vi "Example Remote Callback.vi"() -> ()   [LabVIEW 2013]
uses:
  C:/tf/play/labview/Tinkerforge.dll
  Tinkerforge.dll
panel:
  out "repeats":i32
  out "switchTo":i32
  out "receiverCode":u8
  out "houseCode":u8
  in  "stop":bool
  in  "uid":string="abc"
  in  "port":i32=4223
  in  "host":string="localhost"
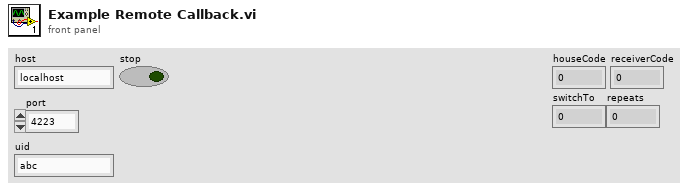
[diagram p1: front panel]
types:
  T1 = cluster{"houseCode":u8, "receiverCode":u8, "repeats":i32, "switchTo":i32}
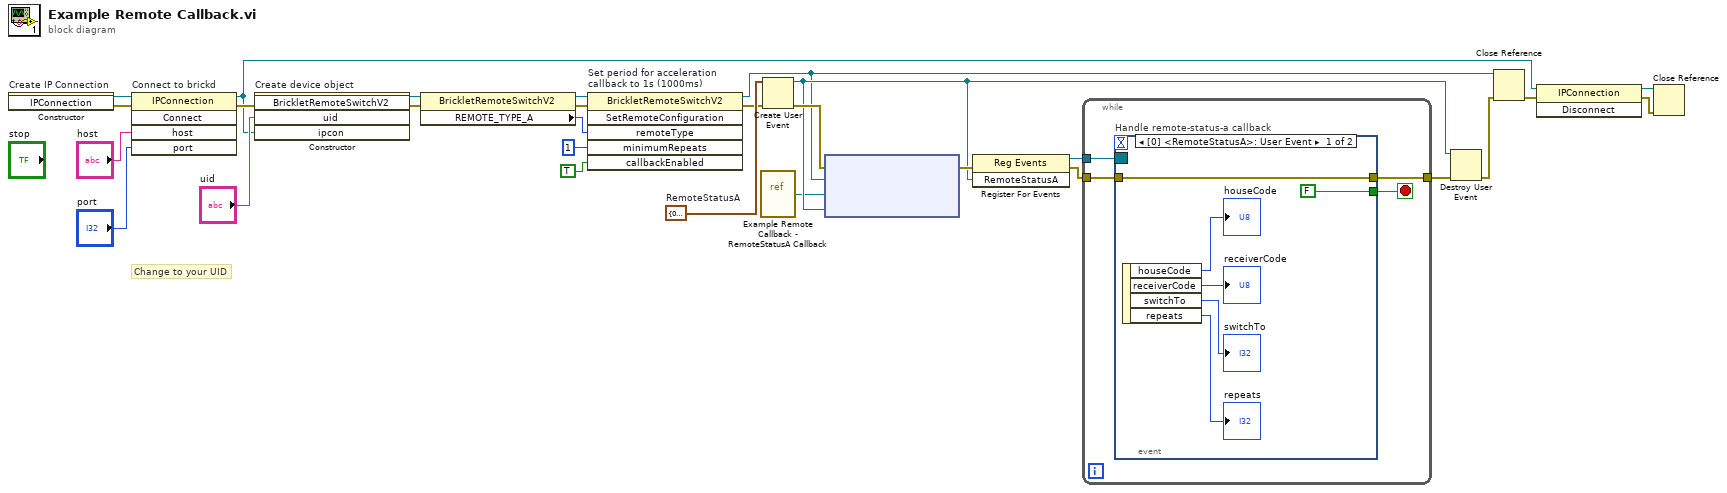
[diagram p0: block diagram]
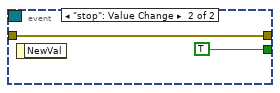
[diagram p2: hidden frame]
diagram:
  w12 = T1 {"houseCode"=0, "receiverCode"=0, "repeats"=0, "switchTo"=0}  # RemoteStatusA
  # "Change to your UID"
  n1 = constructor on="Create IP Connection" class="IPConnection"() -> (reference out=w28:refnum<k24>, error out=w9:errorcluster)  [unwired: 3 in, 1 out]
  n2 = invoke on="Connect to brickd" class="IPConnection" method="Connect"(reference=w28, error in=w9, "host"="host", "port"="port") -> (reference out=w21:refnum<k24>, error out=w24:errorcluster)  [unwired: 1 in, 3 out]
  n3 = constructor on="Create device object" class="BrickletRemoteSwitchV2"(error in=w24, "uid"="uid", "ipcon"=w21) -> (reference out=w8:refnum<k24>, error out=w7:errorcluster)  [unwired: 2 in, 3 out]
  n4 = property class="BrickletRemoteSwitchV2"(reference=w8, error in=w7) -> (reference out=w5:refnum<k24>, error out=w6:errorcluster, "REMOTE_TYPE_A"=w4:u8)
  n5 = invoke on="Set period for acceleration\ncallback to 1s (1000ms)" class="BrickletRemoteSwitchV2" method="SetRemoteConfiguration"(reference=w5, error in=w6, "remoteType"=w4, "minimumRepeats"=1, "callbackEnabled"=TRUE) -> (reference out=w10:refnum<k24>, error out=w11:errorcluster)  [unwired: 1 in, 4 out]
  n6 = vi-ref "Example Remote Callback - RemoteStatusA Callback.vi"() -> ("vi reference"=w1:refnum<vi>)
  n7 = Create User Event(user event datatype=w12, error in=w11) -> (user event=w14:refnum<user-event>, error out=w19:errorcluster)
  n8 = node ("Register Event Callback")(w19, w10, w1, w14) -> (w18:errorcluster)  [unwired: 1 in, 1 out]
  n9 = register-events(error in=w18, w14) -> (reference out=w17:refnum<event-registration>, error out=w15:errorcluster)  [unwired: 1 in]
  n10 = while {
    tunnel: w17 -> [w32]
    tunnel: [w31] -> w16
    tunnel: w15 -> [w30]
    stop <- w29 stop-if-true
    n11 = event "Handle remote-status-a callback" shown="[0] <RemoteStatusA>: User Event" {
      selector: w32 -> [_ _]
      dyn-events: _ -> [_ _]
      timeout: _ -> [_ _]
      tunnel: [w38 w39] -> w31
      tunnel: w30 -> [w38 w39]
      tunnel: [FALSE TRUE] -> w29
      event User Event {
        n12 = event-data() -> ("houseCode"=→"houseCode":u8, "receiverCode"=→"receiverCode":u8, "switchTo"=→"switchTo":i32, "repeats"=→"repeats":i32)  [unwired: 1 in]
      }
      event "stop": Value Change {
        n13 = event-data() -> ()  [unwired: 1 in, 1 out]
      }
    }
  }
  n14 = Destroy User Event(user event=w14, error in=w16) -> (error out=w13:errorcluster)
  n15 = Close Reference(reference=w10, error in (no error)=w13) -> (error out=w23:errorcluster)
  n16 = invoke class="IPConnection" method="Disconnect"(reference=w21, error in=w23) -> (reference out=w20:refnum<k24>, error out=w22:errorcluster)  [unwired: 1 in, 1 out]
  n17 = Close Reference(reference=w20, error in (no error)=w22) -> ()  [unwired: 1 out]
